vi "Big Temp Display.vi"() -> ()   [LabVIEW 2020]
panel:
  out "Red Chart":dbl(graph)
  out "Red and Green Chart":cluster{dbl, dbl}(graph)
  out "Green Chart":dbl(graph)
  out "Tab Control":enum32{"Display", "Configure"}(tab)
  in  "Pause":bool
  in  "Clear Data":bool
  in  "stop":bool
  in  "Configure Button":bool
  out "Readout  Red":dbl format="%_3f"
  out "Readout Green":dbl format="%_3f"
  in  "Alarm Low Green?":bool
  in  "Alarm Low Green":dbl
  in  "Alarm Hi Green?":bool
  in  "Alarm Hi Green":dbl
  in  "Show Data on Chart? Green":bool
  in  "Display What Units? Green":enum32{"Current Temperature", "Rate of Change"}(radio)
  in  "Read Which Value?   Green":enum32{"Sorb", "1K Pot", "He3 Pot", "Probe"}(radio)
  in  "Save Configure":bool
  in  "Alarm Low Red?":bool
  in  "Alarm Low Red":dbl
  in  "Alarm Hi Red?":bool
  in  "Alarm Hi Red":dbl
  in  "Show Data on Chart? Red":bool
  in  "Display What Units? Red":enum32{"Current Temperature", "Rate of Change"}(radio)
  in  "Read Which Value?   Red":enum32{"Sorb", "1K Pot", "He3 Pot", "Probe"}(radio)
  in  "Instrument Address":refnum<visa-resource-name>
  out "error out":errorcluster
  # "Red Channel"
  # "Set Alarms"
  # "Alert when above"
  # "Alert when below"
  # "Green Channel"
  # "Set Alarms"
  # "Alert when above"
  # "Alert when below"
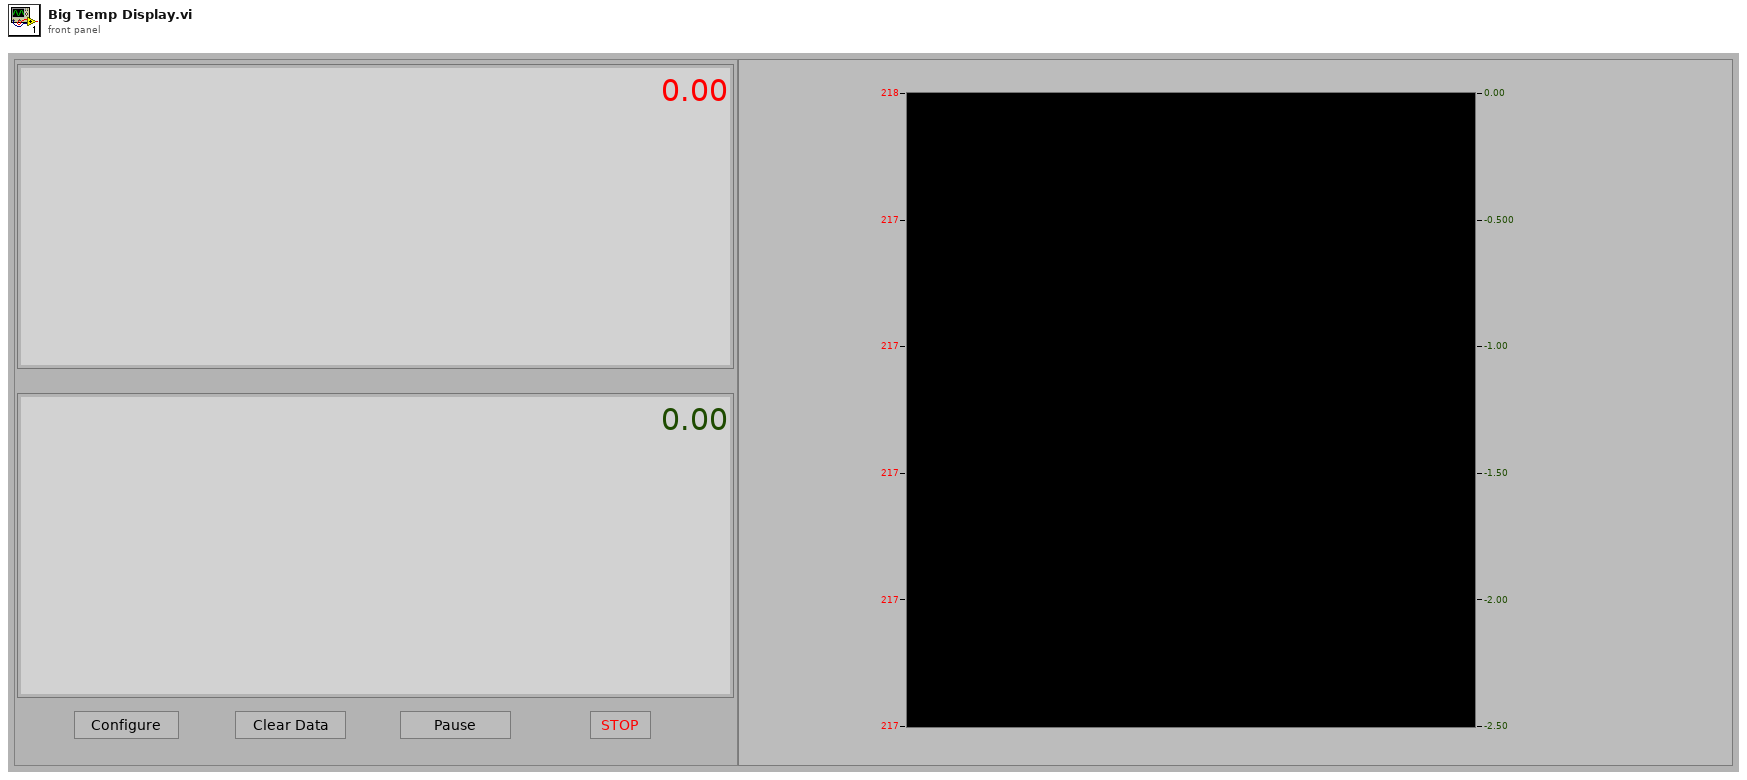
[diagram p1: front panel]
types:
  T1 = cluster{"Read Which Value?   Red":enum32{"Sorb", "1K Pot", "He3 Pot", "Probe"}, "Display What Units? Red":enum32{"Current Temperature", "Rate of Change"}, "Show Data on Chart? Red":bool, "Alarm Hi Red?":bool, "Alarm Hi Red":dbl, "Alarm Low Red?":bool, "Alarm Low Red":dbl}
  T2 = cluster{"Read Which Value?   Green":enum32{"Sorb", "1K Pot", "He3 Pot", "Probe"}, "Display What Units? Green":enum32{"Current Temperature", "Rate of Change"}, "Show Data on Chart? Green":bool, "Alarm Hi Green?":bool, "Alarm Hi Green":dbl, "Alarm Low Green?":bool, "Alarm Low Green":dbl}
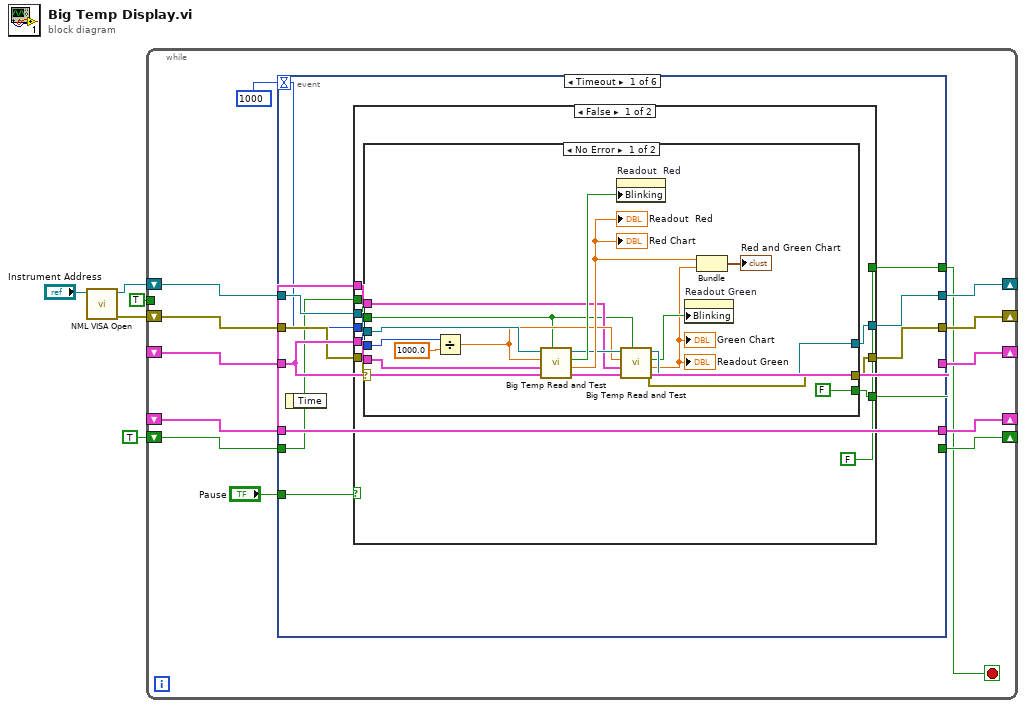
[diagram p0: block diagram]
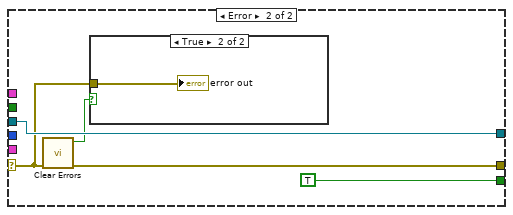
[diagram p2: hidden frame]
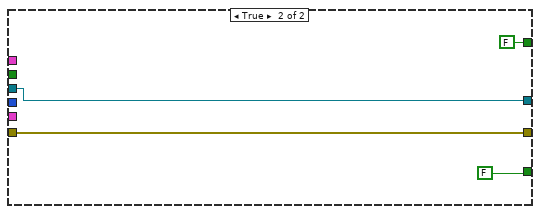
[diagram p4: hidden frame]
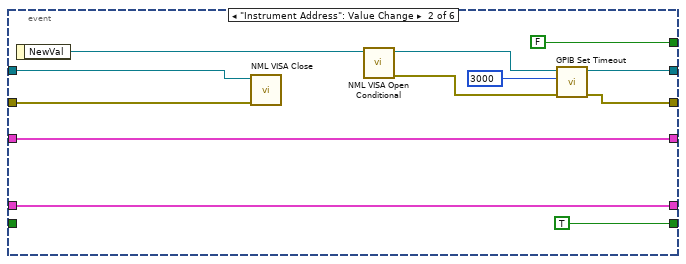
[diagram p5: hidden frame]
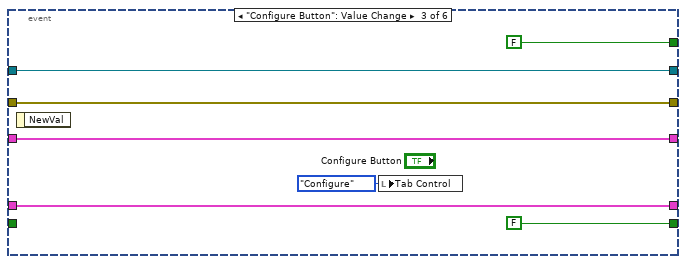
[diagram p6: hidden frame]
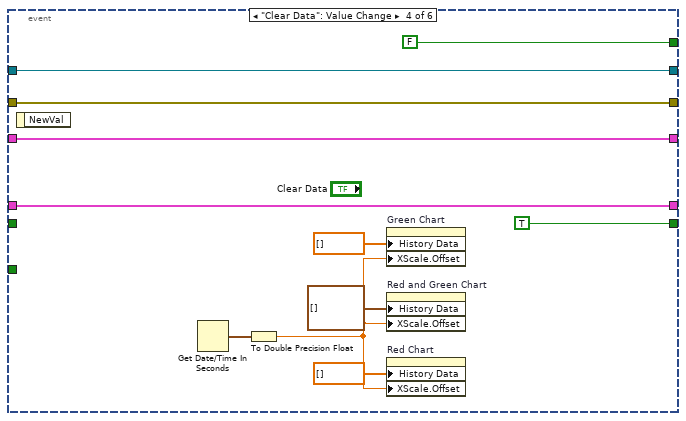
[diagram p7: hidden frame]
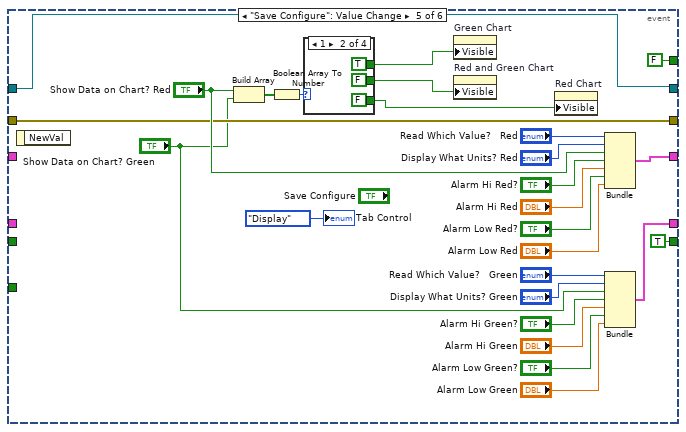
[diagram p8: hidden frame]
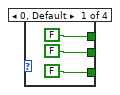
[diagram p9: hidden frame]
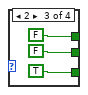
[diagram p10: hidden frame]
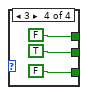
[diagram p11: hidden frame]
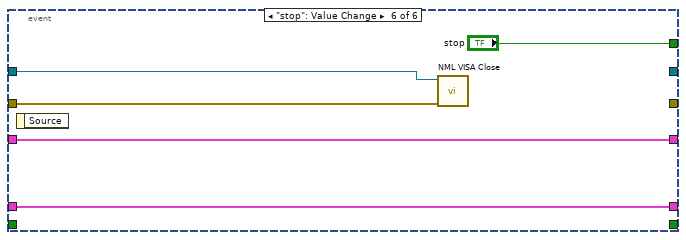
[diagram p12: hidden frame]
diagram:
  n1 = call "NML VISA Open.vi"("VISA resource name"="Instrument Address") -> ("error out"=w3:errorcluster, "VISA resource name out"=w4:refnum<visa-resource-name>)  [unwired: 9 in]
  n2 = while {
    shift-right: [w16] -> _
    shift-left: _ -> [w14]
    shift-right: [w17] -> _
    shift-left: _ -> [w15]
    shift-right: [w12] -> _
    shift-left: w4 -> [w13]
    shift-right: [w10] -> _
    shift-left: w3 -> [w11]
    tunnel: TRUE -> [_]
    shift-right: [w8] -> _
    shift-left: TRUE -> [w9]
    stop <- w7 stop-if-true
    n3 = event shown="[0] Timeout" {
      selector: _ -> [_ _ _ _ _ _]
      dyn-events: _ -> [_ _ _ _ _ _]
      timeout: 1000 -> [w20 _ _ _ _ _]
      tunnel: [w28 w78 w85 w95 w112 w136] -> w17
      tunnel: [w29 w79 w84 w94 w111 w137] -> w16
      tunnel: w15 -> [w28 w78 w85 w95 _ w136]
      tunnel: w14 -> [w29 w79 w84 w94 _ w137]
      tunnel: w13 -> [w25 w76 w82 w90 w102 w139]
      tunnel: [w24 w72 w82 w90 w102 _] -> w12
      tunnel: w11 -> [w27 w77 w83 w89 w103 w138]
      tunnel: [w26 w69 w83 w89 w103 _] -> w10
      tunnel: w9 -> [w22 _ _ _ _ _]
      tunnel: [w23 TRUE FALSE TRUE TRUE _] -> w8
      tunnel: [w21 FALSE ("stop") FALSE ("stop") FALSE ("stop") FALSE ("stop") "stop"] -> w7
      tunnel: "Pause" -> [w19 _ _ _ _ _]
      event Timeout {
        n4 = event-data() -> ()  [unwired: 1 in, 1 out]
        n5 = case shown="False" w19 {
          tunnel: w29 -> [w39 _]
          tunnel: w28 -> [w38 _]
          tunnel: w27 -> [w37 w67]
          tunnel: [w36 w67] -> w26
          tunnel: w25 -> [w35 w65]
          tunnel: [w34 w65] -> w24
          tunnel: [w33 FALSE] -> w23
          tunnel: w22 -> [w32 _]
          tunnel: [FALSE ("stop") FALSE ("stop")] -> w21
          tunnel: w20 -> [w30 _]
          frame False {
            n6 = case shown="No Error" w37 {
              selector: w37 -> [w52 w58]
              tunnel: w39 -> [w46 _]
              tunnel: w38 -> [w55 _]
              tunnel: w35 -> [w53 w62]
              tunnel: [w44 w60] -> w36
              tunnel: [w43 w62] -> w34
              tunnel: [FALSE TRUE] -> w33
              tunnel: w32 -> [w40 _]
              tunnel: w30 -> [w50 _]
              frame No Error {
                n7 = Divide(x=w50, y=1000.0) -> (x/y=w47:dbl)
                n8 = call "Big Temp Read and Test.vi"("Initialize"=w40, "Error In"=w52, "Cluster"=w55, "Cycle Time (S)"=w47, "VISA resource name"=w53) -> ("Error Out"=w45:errorcluster, "Readout"=w49:dbl, "Blinking"=w56:bool, "VISA resource name"=w48:refnum<visa-resource-name>)  [unwired: 3 in]
                "Readout  Red" <- w49
                "Red Chart" <- w49
                n9 = property on="Readout  Red" class="DigNum (strict)"("Blinking"=w56) -> ()  [unwired: 2 in, 2 out]
                n10 = call "Big Temp Read and Test.vi"("Initialize"=w40, "Error In"=w45, "Cluster"=w46, "Cycle Time (S)"=w47, "VISA resource name"=w48) -> ("Error Out"=w44:errorcluster, "Readout"=w41:dbl, "Blinking"=w42:bool, "VISA resource name"=w43:refnum<visa-resource-name>)  [unwired: 3 in]
                "Readout Green" <- w41
                "Green Chart" <- w41
                n11 = property on="Readout Green" class="DigNum (strict)"("Blinking"=w42) -> ()  [unwired: 2 in, 2 out]
                n12 = Bundle("Readout"=w49, "Readout"=w41) -> (→"Red and Green Chart":cluster{"Readout":dbl, "Readout":dbl})  [unwired: 1 in]
              }
              frame Error {
                n13 = call <vilib>:"Clear Errors.vi"("error in (no error)"=w58) -> ("error out"=w60:errorcluster, "specific error cleared?"=w59:bool)  [unwired: 5 in]
                n14 = case shown="True" w59 {
                  tunnel: w58 -> [_ w63]
                  frame False {
                  }
                  frame True {
                    "error out" <- w63
                  }
                }
              }
            }
          }
          frame True {
          }
        }
      }
      event "Instrument Address": Value Change {
        n15 = event-data() -> ("NewVal"=w75:refnum<visa-resource-name>)  [unwired: 1 in]
        n16 = call "NML VISA Close.vi"("Error In"=w77, "VISA resource name"=w76) -> ()  [unwired: 9 in, 1 out]
        n17 = call "NML VISA Open Conditional.vi"("VISA resource name"=w75) -> ("error out"=w70:errorcluster, "dup VISA Session"=w71:refnum<visa-resource-name>)  [unwired: 8 in, 1 out]
        n18 = call "GPIB Set Timeout.vi"("Error In"=w70, "Timeout"=u32 3000, "VISA resource name"=w71) -> ("Error Out"=w69:errorcluster, "dup VISA resource name"=w72:refnum<visa-resource-name>)  [unwired: 2 in, 1 out]
      }
      event "Configure Button": Value Change {
        n19 = event-data() -> ()  [unwired: 1 in, 1 out]
        n20 = local write "Tab Control"(enum32{"Display", "Configure"}."Configure" ("Tab Control")) -> ()
      }
      event "Clear Data": Value Change {
        n21 = event-data() -> ()  [unwired: 1 in, 1 out]
        n22 = Get Date/Time In Seconds() -> (seconds since 1Jan1904=w92:timestamp)
        n23 = To Double Precision Float(number=w92) -> (double precision float=w91:dbl)
        n24 = property on="Green Chart" class="WFChart (strict)"("History Data"=dbl[] [], "XScale.Offset"=w91) -> ()  [unwired: 2 in, 2 out]
        n25 = property on="Red and Green Chart" class="WFChart (strict)"("History Data"=cluster{dbl, dbl}[] [], "XScale.Offset"=w91) -> ()  [unwired: 2 in, 2 out]
        n26 = property on="Red Chart" class="WFChart (strict)"("History Data"=dbl[] [], "XScale.Offset"=w91) -> ()  [unwired: 2 in, 2 out]
      }
      event "Save Configure": Value Change {
        n27 = event-data() -> ()  [unwired: 1 in, 1 out]
        n28 = Build Array("Show Data on Chart? Red", "Show Data on Chart? Green") -> (w99:bool[])
        n29 = Boolean Array To Number(Boolean array=w99) -> (number=w107:u32)
        n30 = case shown="1" w107 {
          tunnel: [FALSE FALSE FALSE TRUE] -> w106
          tunnel: [FALSE TRUE FALSE FALSE] -> w105
          tunnel: [FALSE FALSE TRUE FALSE] -> w104
          frame 0, Default {
          }
          frame 1 {
          }
          frame 2 {
          }
          frame 3 {
          }
        }
        n31 = property on="Green Chart" class="WFChart (strict)"("Visible"=w105) -> ()  [unwired: 2 in, 2 out]
        n32 = property on="Red and Green Chart" class="WFChart (strict)"("Visible"=w106) -> ()  [unwired: 2 in, 2 out]
        n33 = property on="Red Chart" class="WFChart (strict)"("Visible"=w104) -> ()  [unwired: 2 in, 2 out]
        n34 = Bundle("Read Which Value?   Red"="Read Which Value?   Red", "Display What Units? Red"="Display What Units? Red", "Show Data on Chart? Red"="Show Data on Chart? Red", "Alarm Hi Red?"="Alarm Hi Red?", "Alarm Hi Red"="Alarm Hi Red", "Alarm Low Red?"="Alarm Low Red?", "Alarm Low Red"="Alarm Low Red") -> (w112:T1)  [unwired: 1 in]
        n35 = Bundle("Read Which Value?   Green"="Read Which Value?   Green", "Display What Units? Green"="Display What Units? Green", "Show Data on Chart? Green"="Show Data on Chart? Green", "Alarm Hi Green?"="Alarm Hi Green?", "Alarm Hi Green"="Alarm Hi Green", "Alarm Low Green?"="Alarm Low Green?", "Alarm Low Green"="Alarm Low Green") -> (w111:T2)  [unwired: 1 in]
        "Tab Control" <- enum32{"Display", "Configure"}."Display" ("Tab Control")
      }
      event "stop": Value Change {
        n36 = event-data() -> ()  [unwired: 1 in, 1 out]
        n37 = call "NML VISA Close.vi"("Error In"=w138, "VISA resource name"=w139) -> ()  [unwired: 9 in, 1 out]
      }
    }
  }
